vi "Main.vi"(11 "Module Admin":refnum<class "Delacor_lib_QMH_Module Admin.lvclass">) -> ()   [LabVIEW 2025, in "N4L_PSM3750_Interface.lvlib"]
doc: "This template is based from the Queued Message Handler design pattern and the Queued Message Handler Project Template that ships with LabVIEW 2014.\n\nThe main difference is that the Queue is private to this module and communication between modules is done via Broadcast and Request events.\n\nRequest events are wrapped via public API methods and are handled in the Event handler loop in this VI.\nAny module can register for Broadcast events sent by this module.\n\nThe Event Handling Loop generates messages based on user interface actions.\n\nThe Message Handling Loop processes messages generated by the Event Handling Loop, or by other messages. The messages are string values, so new messages can be added easily to the Message Cases case structure in the Message Handling Loop. Each message cluster can also provide an optional value for Message Data, which is a variant that can be converted to whatever message-specific data is required.\n_____\nBased on Delacor QMH Project Template 3.1.0.34.\n\n<b>Note:</b> This VI was modified by the <b>Validate DQMH Module</b> tool to wrap the FP.Open method in the module close code with a Conditional Disable Structure so it does not execute when the Main VI is running as a built EXE.\n\n<b>Note:</b> This VI was modified by the <b>Validate DQMH Module</b> tool to add a call to the Error Reported VI at the end of the 'Exit' MHL frame.\n\n<b>Note:</b> This VI was modified by the <b>Validate DQMH Module</b> tool to call the Release Message Queue VI in the top-level Error case."
uses:
  N4L_PSM3750_Interface.lvlib
  <vilib>/Delacor/Delacor QMH/Libraries/Module Admin_class/Delacor_lib_QMH_Module Admin.lvclass
  <vilib>/MGI/Panel Manager/Panel/Panel/Panel.lvclass
  <vilib>/Utility/miscctls.llb/LVPointTypeDef.ctl
  Module Data--cluster.ctl
  <vilib>/Delacor/Delacor QMH/Libraries/Message Queue_class/Delacor_lib_QMH_Message Queue.lvclass/Delacor_lib_QMH_Message Queue.ctl
  Stop Argument--cluster.ctl
  <vilib>/Delacor/Delacor QMH/Libraries/Module Admin_class/Delacor_lib_QMH_Module Admin.lvclass/Delacor_lib_QMH_Module Admin.ctl
  <vilib>/Delacor/Delacor QMH/Libraries/Message Queue_class/Delacor_lib_QMH_Enqueue Message (Single).vi
  <vilib>/Delacor/Delacor QMH/Libraries/Module Admin_class/Delacor_lib_QMH_Get External Launch.vi
  <vilib>/Utility/error.llb/Error Cluster From Error Code.vi
  <vilib>/ErrorRing/Error Ring.xnode
  <vilib>/Delacor/Delacor QMH/Libraries/Message Queue_class/Delacor_lib_QMH_Message Queue.lvclass
  <vilib>/MGI/Panel Manager/Panel/Panel Helper/Panel Helper.lvclass
  newtons4th-psm17xx-labview-files/NewtonsPSM1735.lvlib
panel:
  out "Connected?":bool
  in  "Panel":refnum<class "Panel.lvclass">
  in  "Simulate MHL Error":bool
  in  "Simulate EHL Error":bool
  out "error out":errorcluster
  out "Status":string
  # "This is a template that creates a DQMH Singleton using the MGI Panel Manager Framwork.\n\nImplement your user interface on this front panel. The Panel Manager Framework will manage showing and hiding the panel in the appropriate spot. \n\nSee the block diagram for more information on how to use this template."
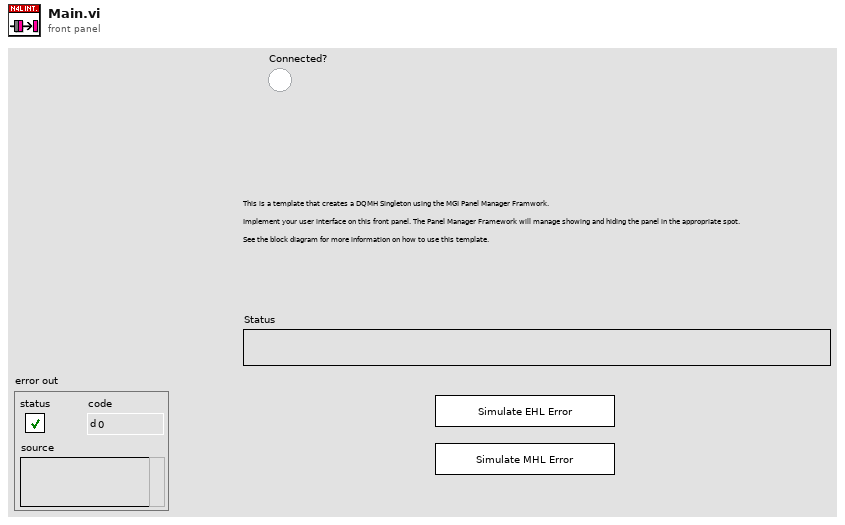
[diagram p1: front panel]
types:
  T1 = typedef "LVPointTypeDef.ctl" = cluster{"Horizontal":i16, "Vertical":i16}
  T2 = typedef "N4L_PSM3750_Interface.lvlib/Request Events--cluster.ctl" = cluster{"Stop Module":refnum<user-event>, "Show Panel":refnum<user-event>, "Hide Panel":refnum<user-event>, "Get Module Execution Status":refnum<user-event>, "Show Diagram":refnum<user-event>, "Change Panel":refnum<user-event>, "Initialise N4L Connection":refnum<user-event>, "Close N4L Connection":refnum<user-event>, "Reset N4L Instrument":refnum<user-event>, "Set Generator Configuration":refnum<user-event>, "Set Generator Output":refnum<user-event>, "Set Range":refnum<user-event>, "Set Trim Configuration":refnum<user-event>}
  T3 = typedef "Panel.lvlib/Panel Helper.lvclass/Panel Events.ctl" = cluster{"My Panel":refnum<user-event>, "Top Level Initialized":refnum<user-event>}
  T4 = typedef "N4L_PSM3750_Interface.lvlib/Module Data--cluster.ctl" = cluster{"Status":string, "State Map":map{string, dbl}}
  T5 = typedef "N4L_PSM3750_Interface.lvlib/Stop Argument--cluster.ctl" = cluster{"Origin":string, "Exit via Stop Module Req?":bool, "Wait for Module to stop?":bool}
  T6 = enum32{"invalid lock state", "Not Locked", "Locked (No Password)", "Password-protected"}
  T7 = typedef "N4L_PSM3750_Interface.lvlib/Initialise--cluster.ctl" = cluster{"VISA resource name":refnum<visa-resource-name>, "Baud Rate":u32, "ID Query":bool, "Reset":bool}
  T8 = typedef "N4L_PSM3750_Interface.lvlib/Generator Config--cluster.ctl" = cluster{"Waveform":enum16{"Sinewave", "Square"}, "Frequency (1000)":dbl, "Amplitude (2)":dbl, "Offset (0)":dbl}
  T9 = typedef "N4L_PSM3750_Interface.lvlib/Range Config--cluster.ctl" = cluster{"Input Ranging Mode (Auto)":enum16{"AUTO", "UPAUTO", "1mV", "3mV", "10mV", "30mV", "100mV", "300mV", "1V", "3V", "10V"}, "Input Input Type (Internal)":u16, "Input Selection (CH1)":enum16{"CH1", "CH2"}, "Input Connection (Main) ":u16, "Input Coupling (Internal)":enum16{"AC+DC", "AC"}, "Input Shunt Value (0,02)":dbl, "Input Voltage Scale factor (1)":dbl}
  T10 = enum16{"AUTO", "UPAUTO", "1mV", "3mV", "10mV", "30mV", "100mV", "300mV", "1V", "3V", "10V"}
  T11 = cluster{"AC Trim Data (Disabled)":u16, "AC Level (1)":dbl, "Tolerance (10)":dbl}
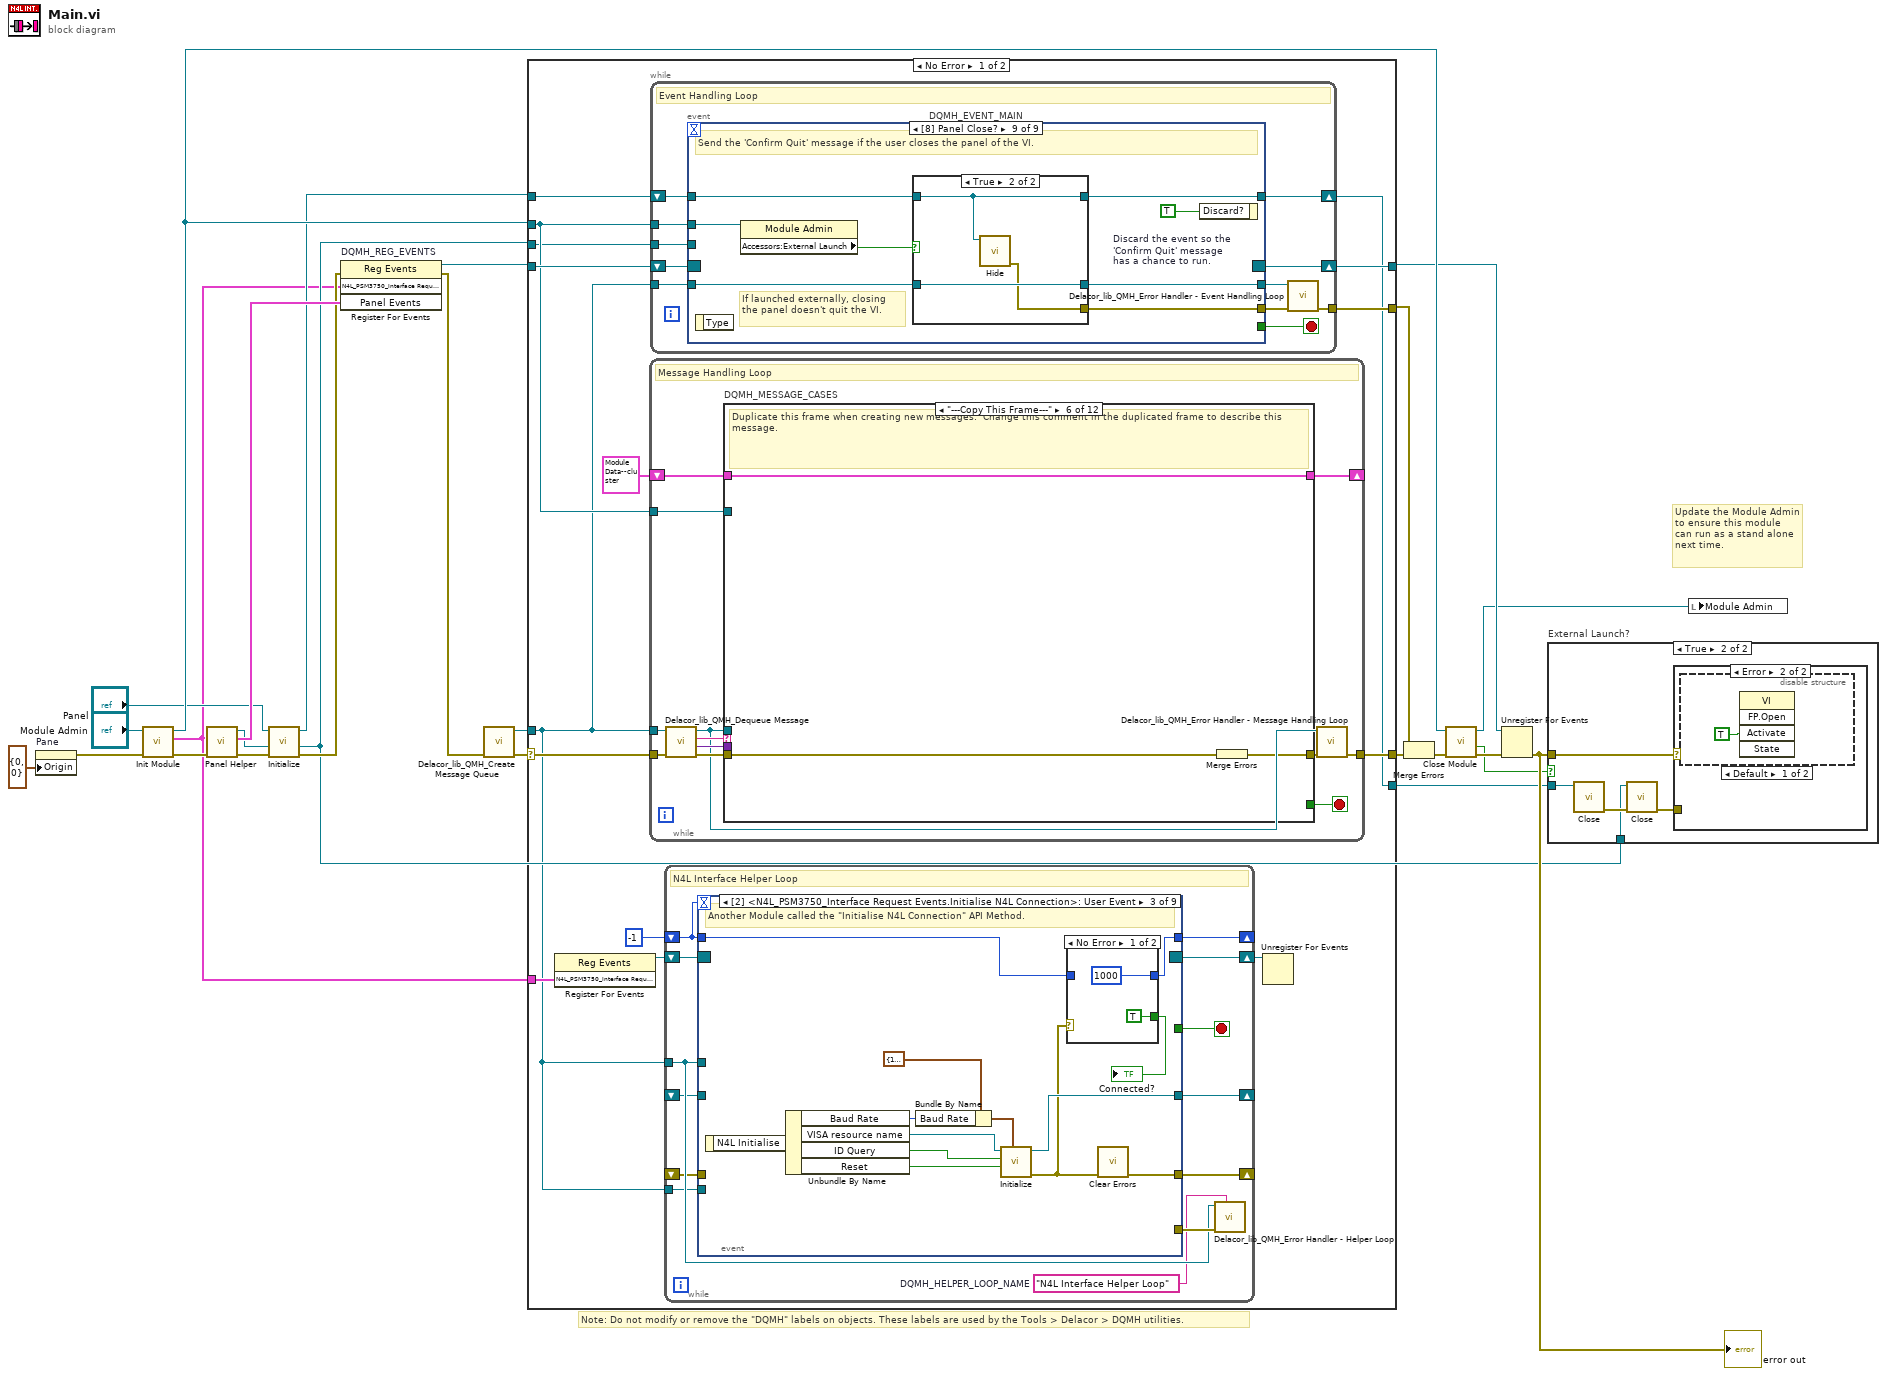
[diagram p0: block diagram]
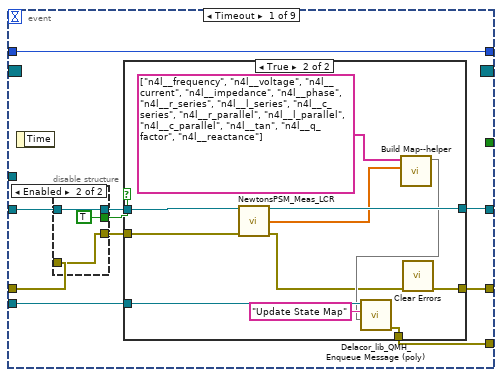
[diagram p5: hidden frame]
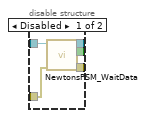
[diagram p6: hidden frame]
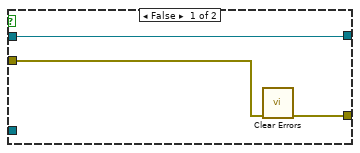
[diagram p7: hidden frame]
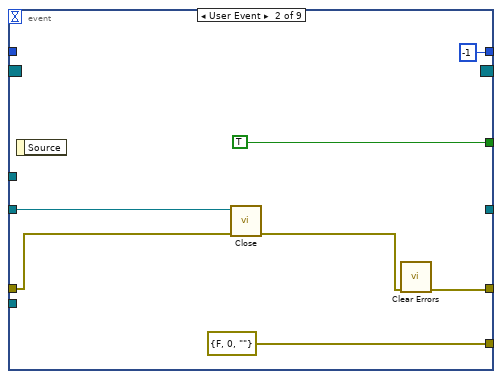
[diagram p8: hidden frame]
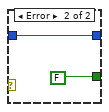
[diagram p9: hidden frame]
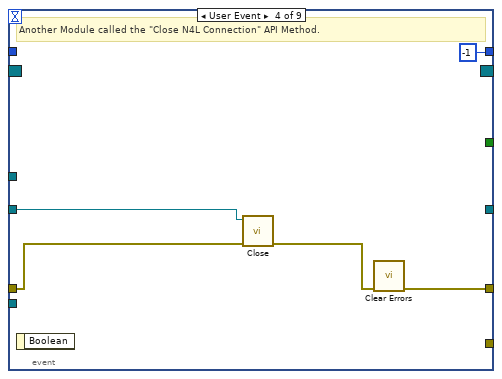
[diagram p10: hidden frame]
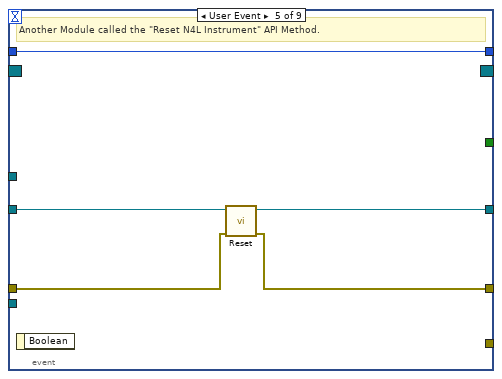
[diagram p11: hidden frame]
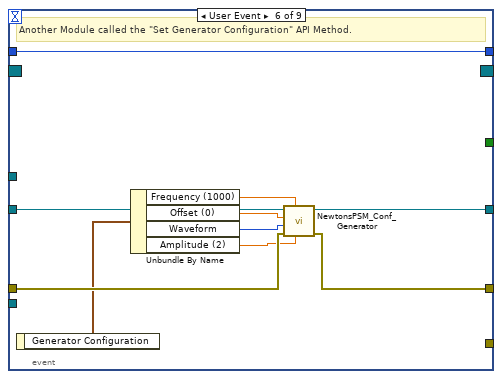
[diagram p12: hidden frame]
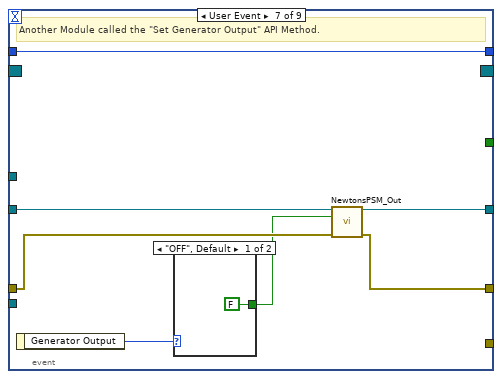
[diagram p13: hidden frame]
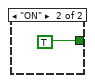
[diagram p14: hidden frame]
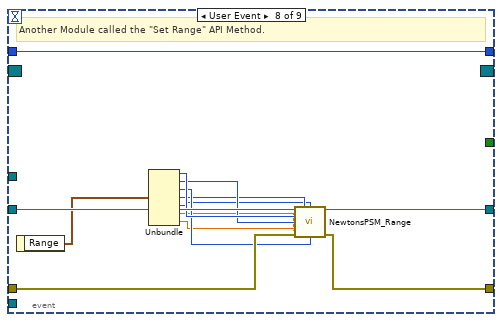
[diagram p15: hidden frame]
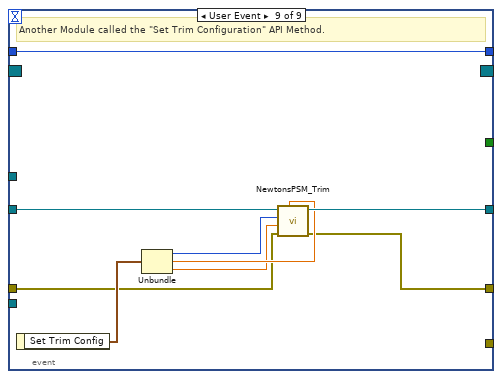
[diagram p16: hidden frame]
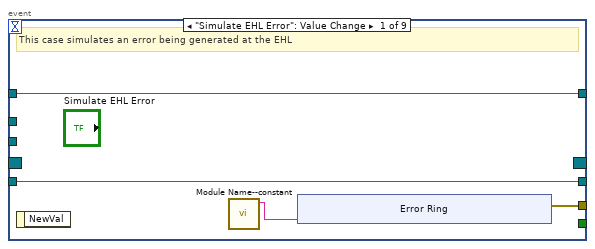
[diagram p17: hidden frame]
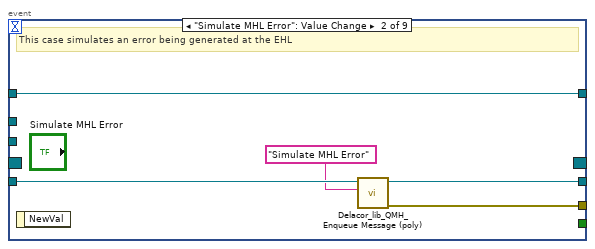
[diagram p18: hidden frame]
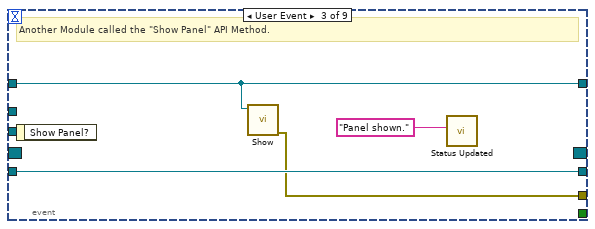
[diagram p19: hidden frame]
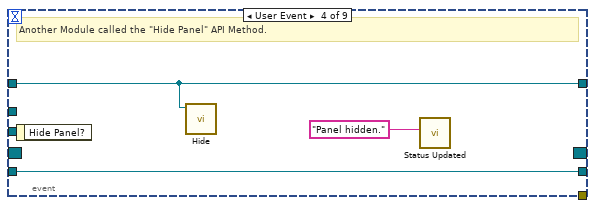
[diagram p20: hidden frame]
diagram:
  # "Note: Do not modify or remove the \"DQMH\" labels on objects. These labels are used by the Tools > Delacor > DQMH utilities."
  # "Update the Module Admin to ensure this module can run as a stand alone next time."
  n1 = property on="Pane" class="Pane"("Origin"=T1 {"Horizontal"=0, "Vertical"=0}) -> (error out=w2:errorcluster)  [unwired: 2 in, 1 out]
  n2 = call "Init Module.vi"("error in (no error)"=w2, "Singleton Module Admin in"="Module Admin") -> ("error out"=w12:errorcluster, "N4L_PSM3750_Interface Request Events"=w1:T2, "Singleton Module Admin out"=w26:refnum<class "Delacor_lib_QMH_Module Admin.lvclass">)  [unwired: 7 in]
  n3 = call <vilib>:"Panel Helper.vi"("Error In"=w12) -> ("Error Out"=w9:errorcluster, "Panel Events"=w11:T3, "Panel Helper out"=w8:refnum<class "Panel Helper.lvclass">)  [unwired: 8 in]
  n4 = call <vilib>:"Initialize.vi"("error in (no error)"=w9, "My Helper in"=w8, "Panel In"="Panel") -> ("error out"=w6:errorcluster, "My Helper out"=w5:refnum<class "Panel Helper.lvclass">, "Panel Out"=w4:refnum<class "Panel.lvclass">)  [unwired: 6 in]
  n5 = register-events "DQMH_REG_EVENTS"(error in=w6, w1, w11) -> (reference out=w23:refnum<event-registration>, error out=w10:errorcluster)  [unwired: 1 in]
  n6 = call <vilib>:"Delacor_lib_QMH_Create Message Queue.vi"("error in"=w10) -> ("error out"=w14:errorcluster, "Message Queue"=w22:refnum<class "Delacor_lib_QMH_Message Queue.lvclass">)  [unwired: 9 in]
  n7 = case shown="No Error" w14 {
    selector: w14 -> [w36 w378]
    tunnel: [w41 w378] -> w25
    tunnel: [w40 w383] -> w24
    tunnel: w23 -> [w38 w383]
    tunnel: w22 -> [w27 w374]
    tunnel: [w37 _] -> w18
    tunnel: w26 -> [w35 w379]
    tunnel: w4 -> [w33 w375]
    tunnel: w5 -> [w34 _]
    tunnel: [w32 w375] -> w13
    tunnel: w1 -> [w31 _]
    frame No Error {
      n8 = register-events ("DQMH_HELPER_REGFOREVENTS")(w31) -> (reference out=w29:refnum<event-registration>)  [unwired: 2 in, 1 out]
      n9 = while {
        tunnel: w27 -> [w246]
        shift-right: [w252] -> _
        shift-left: T4 {"Status"="", "State Map"={}} ("Data Cluster") -> [w253]
        tunnel: w36 -> [w250]
        tunnel: [w244] -> w41
        tunnel: w35 -> [w243]
        stop <- w251 stop-if-true
        # "Message Handling Loop"
        n10 = call-dynamic "Delacor_lib_QMH_Dequeue Message.vi"("error in"=w250, "Message Queue in"=w246) -> ("error out"=w249:errorcluster, "Message Data"=w247:variant, "Message"=w248:string, "Message Queue out"=w245:refnum<class "Delacor_lib_QMH_Message Queue.lvclass">)  [unwired: 6 in]
        n11 = case "DQMH_MESSAGE_CASES" shown="\"---Copy This Frame---\"" w248 {
          selector: w248 -> [_ _ _ _ _ _ _ _ _ _ _ w363]
          tunnel: w245 -> [_ _ _ _ _ _ _ _ w328 w343 w359 _]
          tunnel: w249 -> [w257 w269 w273 w291 w301 w309 w312 w317 w334 w347 w361 _]
          tunnel: [w258 w270 w272 w289 w297 w307 w310 w315 w325 w345 w355 w364] -> w254
          tunnel: w253 -> [w263 w271 w274 w290 w296 w308 w311 w316 w333 w346 w358 w365]
          tunnel: [w262 w271 w274 w290 w295 w308 w311 w316 w333 w346 w358 w365] -> w252
          tunnel: [_ _ _ _ _ _ _ _ _ _ w357 _] -> w251
          tunnel: w247 -> [_ w268 _ _ w300 _ _ _ w332 _ w354 _]
          tunnel: w243 -> [w255 _ _ _ _ _ _ _ w327 _ w348 _]
          frame "Initialize" {
            w261 = "Initial Message" ("Initial Message")
            # "#CodeNeeded - Initialize the appearance of the front panel."
            # "#CodeNeeded - Initialize your state data here."
            # "Initialize - Any operation that needs to be done before the module can receive messages. Synchronize Caller Events.vi will inform Start Module.vi that the module has launched and is ready to receive messages. Module Did Init.vi will broadcast that the module initialized."
            n12 = call "Synchronize Caller Events.vi"("error in (no error)"=w257, "Singleton Module Admin in"=w255) -> ("error out"=w256:errorcluster)  [unwired: 8 in, 1 out]
            n13 = Bundle By Name(cluster=w263, "Status"=w261) -> (w262:T4)
            n14 = local write "Status"(w261) -> ()
            n15 = call "Module Name--constant.vi"() -> ("Module Name"=w259:string)  [unwired: 11 in]
            n16 = call "Module Did Init.vi"("error in (no error)"=w256, "Initialized?"=TRUE, "Origin"=w259) -> ("error out"=w258:errorcluster)  [unwired: 8 in]
          }
          frame "Update Display" {
            # "Broadcast updated status to any VI registered to listen to this module's broadcast events."
            # "Convert the message data to a string to display in the Status indicator."
            # "#CodeRecommended - If you wish to decouple the Message Handling Loop from your user interface, consider creating User Events (like the \"Stop\" event in this VI) to message the Event Handling Loop whenever the user interface needs updating."
            # "Update Display - Update user interface here."
            n17 = Variant To Data(error in=w269, type="" ("Empty String Constant"), Variant=w268) -> (data=w266:string, error out=w265:errorcluster)
            "Status" <- w266
            n18 = call "Status Updated.vi"("error in (no error)"=w265, "Status"=w266) -> ("error out"=w264:errorcluster)  [unwired: 9 in]
            n19 = Merge Errors(w264) -> (w270:errorcluster)
          }
          frame "Show Diagram" {
            # "Show Diagram - Show the block diagram of this VI. Used as a debugging tool. There is a button in the module tester that fires the Show Diagram request, which runs this message. Note that the diagram will not be displayed if it is password-protected and the password is not in the cache."
            n20 = disable-structure shown="RUN_TIME_ENGINE==False" {
              disable-tunnel: [w282 w288] -> w272
              disable-tunnel: w273 -> [w281 w288]
              frame condition #0 (active) {
                # "functionality not available in exe"
                n21 = invoke class="VI" method="Lock State.Get"(error in=w281) -> (error out=w280:errorcluster, "Get Lock State"=w279:T6, "pwd in cache"=w276:bool)  [unwired: 3 in, 1 out]
                n22 = Equal?(x=T6."Password-protected", y=w279) -> (x = y?=w277:bool)
                n23 = Compound Arithmetic op=AND(w277, invert w276) -> (w275:bool)
                n24 = case shown="False" w275 {
                  tunnel: [w285 w287] -> w282
                  tunnel: w280 -> [w283 w287]
                  frame False {
                    n25 = property class="VI"(error in=w283, "BDWin.Open"=TRUE ("Block Diagram Window:Open")) -> (error out=w285:errorcluster)  [unwired: 1 in, 1 out]
                    n26 = call "Status Updated.vi"("Status"="Block Diagram shown." ("format string")) -> ()  [unwired: 10 in, 1 out]
                  }
                  frame True {
                    # "Password-protected VI, and the password is not in the cache. Do not show the diagram."
                  }
                }
              }
              frame condition #1 {
              }
            }
          }
          frame "--- Module Specific ---" {
            # "Separator -- The following cases handle messages specific to this Module."
            n27 = Merge Errors(w291) -> (w289:errorcluster)
          }
          frame "Update State Map" {
            w299 = map{string, dbl} {}  # Size: 0
            n28 = Variant To Data(error in=w301, type=w299, Variant=w300) -> (data=w294:map{string, dbl}, error out=w298:errorcluster)
            n29 = Unbundle By Name(w296) -> ("State Map"=w293:map{string, dbl})
            n30 = for {
              tunnel: w294 -> [w304] mode=indexing
              shift-right: [w305] -> w292
              shift-left: w293 -> [w306]
              n31 = Unbundle(w304) -> (w303:string, w302:dbl)
              n32 = Insert Into Map(map in=w306, key=w303, value=w302) -> (map out=w305:map{string, dbl})  [unwired: 2 out]
            }
            n33 = Bundle By Name(cluster=w296, "State Map"=w292) -> (w295:T4)
            n34 = call "Broadcast State.vi"("error in"=w298, "State Map"=w292) -> ("error out"=w297:errorcluster)  [unwired: 9 in]
          }
          frame "---Copy This Frame---" {
            # "Duplicate this frame when creating new messages.  Change this comment in the duplicated frame to describe this message."
            n35 = Merge Errors(w309) -> (w307:errorcluster)
          }
          frame "--- Exit and Error Handling---" {
            # "Separator - The following cases handle errors and exit messages."
            n36 = Merge Errors(w312) -> (w310:errorcluster)
          }
          frame "Simulate MHL Error" {
            # "Simulate an error occurring at the MHL"
            n37 = call "Module Name--constant.vi"() -> ("Module Name"=w314:string)  [unwired: 11 in]
            n38 = xnode "Error Ring"("parameter 0"=w314) -> ("error out"=w313:errorcluster)
            n39 = Merge Errors(w317, w313) -> (w315:errorcluster)
          }
          frame "Error" {
            # "#CodeRecommended - If you ever change the name of this \"Error\" message, you'll need to update the name in the Check Loop Error.vi as well."
            # "#CodeRecommended - If the module is running in standalone mode (External Launch = FALSE), this code will pop up an error dialog and call the 'Exit' message if an error occurs. Add more fine-grained error handling here."
            # "Error - Check the error message data and respond accordingly. This message is sent by the \"Error Handler\" VIs at the end of each loop in this application."
            n40 = property class="Module Admin"(reference=w327) -> ("Accessors:External Launch"=w326:bool)  [unwired: 1 in, 2 out]
            n41 = Variant To Data(error in=w334, type=errorcluster {"status"=FALSE, "code"=0, "source"=""} ("error constant"), Variant=w332) -> (data=w335:errorcluster, error out=w330:errorcluster)
            n42 = call "Error Reported.vi"("Error"=w335) -> ()  [unwired: 10 in, 1 out]
            n43 = case shown="False" w326 {
              tunnel: [w340 _] -> w329
              tunnel: w328 -> [w339 _]
              tunnel: w335 -> [w336 _]
              frame False {
                # "If the module is running standalone, then pop up an error dialog and call the \"Exit\" message."
                n44 = call <vilib>:"Simple Error Handler.vi"("error in (no error)"=w336) -> ()  [unwired: 4 in, 5 out]
                n45 = call-poly <vilib>:"Delacor_lib_QMH_Enqueue Message (poly).vi"("Priority Message? (F)"=TRUE, "Message"="Exit", "Message Queue in"=w339) -> ("error out"=w340:errorcluster)  [unwired: 7 in, 1 out]
              }
              frame True {
                # "If the module was launched externally, calling the Error Reported broadcast VI is the only action performed by the \"Error\" message. The module's caller can then process the error appropriately."
              }
            }
            n46 = Merge Errors(w330, w329) -> (w325:errorcluster)
            n47 = local write "error out"(w325) -> ()
          }
          frame "Confirm Quit" {
            # "#CodeNeeded - If you want to provide an \"Are you sure\" dialog (or some other notification) before the application exits, place that code here. This message is typically sent from a Panel Close? event."
            # "Confirm Quit - Message that can confirm whether or not the user wants to exit the application."
            n48 = call-poly <vilib>:"Delacor_lib_QMH_Enqueue Message (poly).vi"("Priority Message? (F)"=TRUE, "error in"=w347, "Message"="Exit", "Message Queue in"=w343) -> ("error out"=w344:errorcluster)  [unwired: 6 in, 1 out]
            n49 = Merge Errors(w344) -> (w345:errorcluster)
          }
          frame "Exit" {
            w352 = 91  # 91: not all Exit messages will have an argument
            w357 = TRUE  # Stop the VI
            # "Release the message queue reference"
            # "#CodeNeeded - Add any required cleanup code here"
            # "Exit - Exit the application."
            n50 = Variant To Data(error in=w361, type=T5 {"Origin"="", "Exit via Stop Module Req?"=FALSE, "Wait for Module to stop?"=FALSE} ("Stop Argument"), Variant=w354) -> (data=w350:T5, error out=w353:errorcluster)
            n51 = call <vilib>:"Clear Errors.vi"("error in (no error)"=w353, "specific error code to clear (0: all)"=w352) -> ("error out"=w360:errorcluster)  [unwired: 4 in, 1 out]
            n52 = call-dynamic "Delacor_lib_QMH_Release Message Queue.vi"("error in"=w360, "Message Queue"=w359) -> ("error out"=w356:errorcluster)  [unwired: 9 in]
            n53 = call "Handle Exit.vi"("Stop Argument"=w350, "Admin in"=w348) -> ("error out"=w349:errorcluster)  [unwired: 8 in, 1 out]
            n54 = Merge Errors(w349, w356) -> (w355:errorcluster)
            n55 = call "Error Reported.vi"("Error"=w355) -> ()  [unwired: 10 in, 1 out]
          }
          frame Default {
            # "'Default' case only runs if there is a message that isn't defined in any of the other cases.  Output a programming error."
            n56 = call "Module Name--constant.vi"() -> ("Module Name"=w362:string)  [unwired: 11 in]
            n57 = xnode "Error Ring"("parameter 0"=w363, "parameter 1"=w362) -> ("error out"=w364:errorcluster)
          }
        }
        n58 = call-dynamic "Delacor_lib_QMH_Error Handler - Message Handling Loop.vi"("error in"=w254, "Message Queue in"=w245) -> ("dup error in"=w244:errorcluster)  [unwired: 8 in, 1 out]
      }
      n59 = while {
        tunnel: w27 -> [w172]
        shift-right: [w170] -> w40
        shift-left: w38 -> [w171]
        tunnel: [w166] -> w37
        tunnel: w35 -> [w165]
        tunnel: w34 -> [w164]
        shift-right: [w162] -> w32
        shift-left: w33 -> [w163]
        stop <- w168 stop-if-true
        # "Event Handling Loop"
        n60 = event "DQMH_EVENT_MAIN" shown="[8] Panel Close?" {
          selector: w171 -> [_ _ _ _ _ _ _ _ _]
          dyn-events: [_ _ _ _ _ _ _ _ _] -> w170
          timeout: _ -> [_ _ _ _ _ _ _ _ _]
          tunnel: [_ _ _ _ _ _ TRUE ("Discard?") _ _] -> w168
          tunnel: w172 -> [w176 w188 w192 w195 w199 w204 w216 w226 w233]
          tunnel: [w175 w185 w190 _ w198 w201 w210 w222 w232] -> w169
          tunnel: [w176 w187 w192 w195 w199 w203 w215 w226 w231] -> w167
          tunnel: w165 -> [_ _ _ _ _ _ _ _ w230]
          tunnel: w164 -> [_ _ _ _ _ _ _ w221 _]
          tunnel: w163 -> [w173 w184 w191 w194 w196 w200 w205 w225 w228]
          tunnel: [w173 w184 w191 w194 w196 w200 w205 w220 w227] -> w162
          event "Simulate EHL Error": Value Change {
            # "This case simulates an error being generated at the EHL"
            n61 = event-data() -> ()  [unwired: 1 in, 1 out]
            n62 = call "Module Name--constant.vi"() -> ("Module Name"=w174:string)  [unwired: 11 in]
            n63 = xnode "Error Ring"("parameter 0"=w174) -> ("error out"=w175:errorcluster)
          }
          event "Simulate MHL Error": Value Change {
            # "This case simulates an error being generated at the EHL"
            n64 = event-data() -> ()  [unwired: 1 in, 1 out]
            n65 = call-poly <vilib>:"Delacor_lib_QMH_Enqueue Message (poly).vi"("Message"="Simulate MHL Error", "Message Queue in"=w188) -> ("error out"=w185:errorcluster, "Message Queue out"=w187:refnum<class "Delacor_lib_QMH_Message Queue.lvclass">)  [unwired: 8 in]
          }
          event User Event {
            # "Another Module called the \"Show Panel\" API Method."
            n66 = event-data() -> ()  [unwired: 1 in, 1 out]
            n67 = call <vilib>:"Show.vi"("Panel in"=w191) -> ("Error Out"=w190:errorcluster)  [unwired: 10 in]
            n68 = call "Status Updated.vi"("Status"="Panel shown." ("format string")) -> ()  [unwired: 10 in, 1 out]
          }
          event User Event {
            # "Another Module called the \"Hide Panel\" API Method."
            n69 = event-data() -> ()  [unwired: 1 in, 1 out]
            n70 = call <vilib>:"Hide.vi"("Panel In"=w194) -> ()  [unwired: 10 in, 1 out]
            n71 = call "Status Updated.vi"("Status"="Panel hidden." ("format string")) -> ()  [unwired: 10 in, 1 out]
          }
          event User Event {
            # "Another Module called the \"Get Module Execution Status\" API Method."
            n72 = event-data() -> ()  [unwired: 1 in, 1 out]
            n73 = call "Update Module Execution Status.vi"("Running?"=TRUE) -> ("error out"=w198:errorcluster)  [unwired: 10 in]
          }
          event User Event {
            # "Another Module called the \"Show Diagram\" API Method."
            n74 = event-data() -> ()  [unwired: 1 in, 1 out]
            n75 = call-poly <vilib>:"Delacor_lib_QMH_Enqueue Message (poly).vi"("Message"="Show Diagram", "Message Queue in"=w204) -> ("error out"=w201:errorcluster, "Message Queue out"=w203:refnum<class "Delacor_lib_QMH_Message Queue.lvclass">)  [unwired: 8 in]
          }
          event User Event {
            # "The Stop Module Event can get fired from the Exit message in the MHL. The queue gets destroyed in that case. If the queue no longer exists, the Enqueue Exit as a priority message will return error 1. It is safe to ignore, because the module is already exiting."
            # "Another Module called the \"Stop Module\" API Method  or the Message Handling Loop below."
            n76 = event-data() -> ("Origin"=w214:string, "Exit via Stop Module Req?"=w208:bool, "Wait for Module to stop?"=w207:bool)  [unwired: 1 in]
            n77 = call <vilib>:"Hide.vi"("Panel In"=w205) -> ()  [unwired: 10 in, 1 out]
            n78 = local write "Status"(w214) -> ()
            n79 = Bundle By Name(cluster=T5 {"Origin"="", "Exit via Stop Module Req?"=FALSE, "Wait for Module to stop?"=FALSE} ("Stop Argument"), "Exit via Stop Module Req?"=w208, "Wait for Module to stop?"=w207) -> (w206:T5)
            n80 = call-poly <vilib>:"Delacor_lib_QMH_Enqueue Message (poly).vi"("Priority Message? (F)"=TRUE, "Message Data"=w206, "Message"="Exit", "Message Queue in"=w216) -> ("error out"=w211:errorcluster, "Message Queue out"=w215:refnum<class "Delacor_lib_QMH_Message Queue.lvclass">)  [unwired: 6 in]
            n81 = call <vilib>:"Clear Errors.vi"("error in (no error)"=w211, "specific error code to clear (0: all)"=1) -> ("error out"=w210:errorcluster)  [unwired: 4 in, 1 out]
          }
          event User Event {
            # "Another Module called the \"Change Panel\" API Method."
            n82 = event-data() -> ("New Panel"=w224:refnum<class "Panel.lvclass">)  [unwired: 1 in]
            n83 = call-dynamic <vilib>:"Close.vi"("Panel In"=w225) -> ("Error Out"=w223:errorcluster)  [unwired: 10 in]
            n84 = call <vilib>:"Initialize.vi"("error in (no error)"=w223, "My Helper in"=w221, "Panel In"=w224) -> ("error out"=w222:errorcluster, "Panel Out"=w220:refnum<class "Panel.lvclass">)  [unwired: 6 in, 1 out]
            n85 = call "Status Updated.vi"("Status"="Panel changed.") -> ()  [unwired: 10 in, 1 out]
          }
          event Panel Close? {
            w234 = TRUE  # Discard the event so the 'Confirm Quit' message has a chance to run.
            # "If launched externally, closing the panel doesn't quit the VI."
            # "Send the 'Confirm Quit' message if the user closes the panel of the VI."
            n86 = event-data() -> ()  [unwired: 1 in, 1 out]
            n87 = property class="Module Admin"(reference=w230) -> ("Accessors:External Launch"=w229:bool)  [unwired: 1 in, 2 out]
            n88 = case shown="True" w229 {
              tunnel: w233 -> [w239 w242]
              tunnel: [w238 w240] -> w232
              tunnel: [w237 w242] -> w231
              tunnel: w228 -> [w235 w241]
              tunnel: [w235 w241] -> w227
              frame False {
                n89 = call-poly <vilib>:"Delacor_lib_QMH_Enqueue Message (poly).vi"("Message"="Confirm Quit", "Message Queue in"=w239) -> ("error out"=w238:errorcluster, "Message Queue out"=w237:refnum<class "Delacor_lib_QMH_Message Queue.lvclass">)  [unwired: 8 in]
              }
              frame True {
                n90 = call <vilib>:"Hide.vi"("Panel In"=w241) -> ("Error Out"=w240:errorcluster)  [unwired: 10 in]
              }
            }
            n91 = event-data("Discard?"=w234) -> ()  [unwired: 1 in, 1 out]
          }
        }
        n92 = call-dynamic "Delacor_lib_QMH_Error Handler - Event Handling Loop.vi"("error in"=w169, "Message Queue in"=w167) -> ("dup error in"=w166:errorcluster)  [unwired: 8 in, 1 out]
      }
      n93 = while "DQMH_HELPER_LOOP" {
        shift-right: [w54] -> _
        shift-left: -1 -> [w53]
        shift-right: [w51] -> w30
        shift-left: w29 -> [w52]
        tunnel: w27 -> [w48]
        shift-right: [w46] -> _
        shift-left: _ -> [w45]
        shift-right: [w44] -> _
        shift-left: _ -> [w43]
        tunnel: w27 -> [w42]
        stop <- w50 stop-if-true
        w47 = "N4L Interface Helper Loop"  # DQMH_HELPER_LOOP_NAME
        # "N4L Interface Helper Loop"
        n94 = event "DQMH_HELPER_EVENT_STRUCTURE" shown="[2] <N4L_PSM3750_Interface Request Events.Initialise N4L Connection>: User Event" {
          selector: w52 -> [_ _ _ _ _ _ _ _ _]
          dyn-events: [_ _ _ _ _ _ _ _ _] -> w51
          timeout: w53 -> [_ _ _ _ _ _ _ _ _]
          tunnel: w53 -> [w64 _ w98 _ w120 w130 w137 w152 w161]
          tunnel: [w64 -1 w97 -1 w120 w130 w137 w152 w161] -> w54
          tunnel: [_ TRUE _ _ _ _ _ _ _] -> w50
          tunnel: [w57 errorcluster {"status"=FALSE, "code"=0, "source"=""} ("error constant") _ _ _ _ _ _ _] -> w49
          tunnel: w48 -> [_ _ _ _ _ _ _ _ _]
          tunnel: [w56 w88 w95 w111 w117 w127 w134 w148 w153] -> w46
          tunnel: w45 -> [w62 w90 _ w114 w116 w126 w133 w149 w154]
          tunnel: [w59 _ w99 _ w118 w128 w135 w150 w159] -> w44
          tunnel: w43 -> [w63 w91 _ w115 w119 w129 w136 w151 w160]
          tunnel: w42 -> [w58 _ _ _ _ _ _ _ _]
          event Timeout {
            n95 = event-data() -> ()  [unwired: 1 in, 1 out]
            n96 = disable-structure shown="Enabled" {
              disable-tunnel: w63 -> [w69 w72]
              disable-tunnel: w62 -> [w68 w70]
              disable-tunnel: [w67 w72] -> w61
              disable-tunnel: [w66 w70] -> w60
              disable-tunnel: [w65 TRUE ("Data Available")] -> w55
              frame Disabled {
                n97 = call "NewtonsPSM_WaitData.vi"("error in (no error)"=w68, "VISA session"=w69) -> ("error out"=w66:errorcluster, "Data Available"=w65:bool, "dup VISA session"=w67:refnum<visa-resource-name>)  [unwired: 5 out]
              }
              frame Enabled {
              }
            }
            n98 = case shown="True" w55 {
              tunnel: w61 -> [w75 w86]
              tunnel: w60 -> [w73 w85]
              tunnel: [w75 w84] -> w59
              tunnel: w58 -> [_ w81]
              tunnel: [_ w80] -> w57
              tunnel: [w74 w76] -> w56
              frame False {
                n99 = call <vilib>:"Clear Errors.vi"("error in (no error)"=w73) -> ("error out"=w74:errorcluster)  [unwired: 5 in, 1 out]
              }
              frame True {
                n100 = call "NewtonsPSM_Meas_LCR.vi"("VISA session"=w86, "error in (no error)"=w85) -> ("dup VISA session"=w84:refnum<visa-resource-name>, "Measure"=w83:dbl[], "error out"=w77:errorcluster)  [unwired: 10 in, 1 out]
                n101 = call "Build Map--helper.vi"("Measure"=w83, "Array"=string[] ["n4l__frequency", "n4l__voltage", "n4l__current", "n4l__impedance", "n4l__phase", "n4l__r_series", "n4l__l_series", "n4l__c_series", "n4l__r_parallel", "n4l__l_parallel", "n4l__c_parallel", "n4l__tan", "n4l__q_factor", "n4l__reactance"]) -> ("Map"=w78:map{string, dbl})  [unwired: 9 in]
                n102 = call-poly <vilib>:"Delacor_lib_QMH_Enqueue Message (poly).vi"("Message Data"=w78, "Message"="Update State Map", "Message Queue in"=w81) -> ("error out"=w80:errorcluster)  [unwired: 7 in, 1 out]
                n103 = call <vilib>:"Clear Errors.vi"("error in (no error)"=w77) -> ("error out"=w76:errorcluster)  [unwired: 5 in, 1 out]
              }
            }
          }
          event User Event {
            n104 = event-data() -> ()  [unwired: 1 in, 1 out]
            n105 = call <vilib>:"Close.vi"("error in (no error)"=w90, "VISA resource name"=w91) -> ("error out"=w87:errorcluster)  [unwired: 9 out]
            n106 = call <vilib>:"Clear Errors.vi"("error in (no error)"=w87) -> ("error out"=w88:errorcluster)  [unwired: 5 in, 1 out]
          }
          event User Event {
            # "Another Module called the \"Initialise N4L Connection\" API Method."
            n107 = event-data() -> ("N4L Initialise"=w106:T7)  [unwired: 1 in]
            n108 = Unbundle By Name(w106) -> ("Baud Rate"=w103:u32, "VISA resource name"=w105:refnum<visa-resource-name>, "ID Query"=w101:bool, "Reset"=w100:bool)
            n109 = Bundle By Name(cluster=cluster{"Baud Rate":u32} {"Baud Rate"=19200} ("Serial Configuration"), "Baud Rate"=w103) -> (w102:cluster{"Baud Rate":u32})
            n110 = call <vilib>:"Initialize.vi"("Serial Configuration"=w102, "Reset (True)"=w100, "ID Query (True)"=w101, "VISA resource name"=w105) -> ("error out"=w96:errorcluster, "VISA resource name out"=w99:refnum<visa-resource-name>)  [unwired: 6 in]
            n111 = case shown="No Error" w96 {
              tunnel: w98 -> [_ w110]
              tunnel: [1000 w110] -> w97
              tunnel: [TRUE FALSE] -> w94
              frame No Error {
              }
              frame Error {
              }
            }
            "Connected?" <- w94
            n112 = call <vilib>:"Clear Errors.vi"("error in (no error)"=w96) -> ("error out"=w95:errorcluster)  [unwired: 5 in, 1 out]
          }
          event User Event {
            # "Another Module called the \"Close N4L Connection\" API Method."
            n113 = event-data() -> ()  [unwired: 1 in, 1 out]
            n114 = call <vilib>:"Close.vi"("error in (no error)"=w114, "VISA resource name"=w115) -> ("error out"=w112:errorcluster)  [unwired: 9 in]
            n115 = call <vilib>:"Clear Errors.vi"("error in (no error)"=w112) -> ("error out"=w111:errorcluster)  [unwired: 5 in, 1 out]
          }
          event User Event {
            # "Another Module called the \"Reset N4L Instrument\" API Method."
            n116 = event-data() -> ()  [unwired: 1 in, 1 out]
            n117 = call "Reset.vi"("error in (no error)"=w116, "VISA resource name"=w119) -> ("error out"=w117:errorcluster, "VISA resource name out"=w118:refnum<visa-resource-name>)  [unwired: 8 in]
          }
          event User Event {
            # "Another Module called the \"Set Generator Configuration\" API Method."
            n118 = event-data() -> ("Generator Configuration"=w125:T8)  [unwired: 1 in]
            n119 = Unbundle By Name(w125) -> ("Frequency (1000)"=w121:dbl, "Offset (0)"=w122:dbl, "Waveform"=w124:enum16{"Sinewave", "Square"}, "Amplitude (2)"=w123:dbl)
            n120 = call "NewtonsPSM_Conf_Generator.vi"("Amplitude (2)"=w123, "Frequency (1000)"=w121, "error in"=w126, "Waveform (Sinewave)"=w124, "Offset (0)"=w122, "VISA.name"=w129) -> ("error out"=w127:errorcluster, "VISA.name out"=w128:refnum<visa-resource-name>)  [unwired: 4 in]
          }
          event User Event {
            # "Another Module called the \"Set Generator Output\" API Method."
            n121 = event-data() -> ("Generator Output"=w132:enum16{"OFF", "ON"})  [unwired: 1 in]
            n122 = case shown="\"OFF\", Default" w132 {
              tunnel: [FALSE TRUE] -> w131
              frame "OFF", Default {
              }
              frame "ON" {
              }
            }
            n123 = call "NewtonsPSM_Out.vi"("VISA session"=w136, "Output (F: OFF)"=w131, "error in (no error)"=w133) -> ("dup VISA session"=w135:refnum<visa-resource-name>, "error out"=w134:errorcluster)  [unwired: 11 in]
          }
          event User Event {
            # "Another Module called the \"Set Range\" API Method."
            n124 = event-data() -> ("Range"=w147:T9)  [unwired: 1 in]
            n125 = Unbundle(w147) -> ("Input Ranging Mode (Auto)"=w146:T10, "Input Input Type (Internal)"=w145:u16, "Input Selection (CH1)"=w144:enum16{"CH1", "CH2"}, "Input Connection (Main)"=w143:u16, "Input Coupling (Internal)"=w142:enum16{"AC+DC", "AC"}, "Input Shunt Value (0,02)"=w140:dbl, "Input Voltage Scale factor (1)"=w141:dbl)
            n126 = call "NewtonsPSM_Range.vi"("VISA session"=w151, "Input Connection (Main)"=w143, "Input Coupling (Internal)"=w142, "Input Ranging Mode (Auto)"=w146, "Input Input Type (Internal)"=w145, "Input Voltage Scale factor (1)"=w141, "error in (no error)"=w149, "Input Shunt Value (0,02)"=w140, "Input Selection (CH1)"=w144) -> ("dup VISA session"=w150:refnum<visa-resource-name>, "error out"=w148:errorcluster)  [unwired: 5 in]
          }
          event User Event {
            # "Another Module called the \"Set Trim Configuration\" API Method."
            n127 = event-data() -> ("Set Trim Config"=w158:T11)  [unwired: 1 in]
            n128 = Unbundle(w158) -> ("AC Trim Data (Disabled)"=w157:u16, "AC Level (1)"=w156:dbl, "Tolerance (10)"=w155:dbl)
            n129 = call "NewtonsPSM_Trim.vi"("AC Level (1)"=w156, "error in"=w154, "Tolerance (10)"=w155, "AC Trim Data (Disabled)"=w157, "VISA.name"=w160) -> ("error out"=w153:errorcluster, "VISA.name out"=w159:refnum<visa-resource-name>)  [unwired: 5 in]
          }
        }
        n130 = call-dynamic "Delacor_lib_QMH_Error Handler - Helper Loop.vi"("Error Debug"=w47, "error in"=w49, "Message Queue in"=w48) -> ()  [unwired: 7 in, 2 out]
      }
      n131 = Unregister For Events(event registration refnum=w30) -> ()  [unwired: 1 in, 1 out]
    }
    frame Error {
      # "Synchronize Caller Events.vi will inform Start Module.vi that the module has launched and will let the code calling Start Module.vi register for broadcasts and would permit the caller receive the broadcast that an error occurred at launch time."
      n132 = call-dynamic "Delacor_lib_QMH_Release Message Queue.vi"("Message Queue"=w374) -> ()  [unwired: 10 in, 1 out]
      n133 = call "Synchronize Caller Events.vi"("Singleton Module Admin in"=w379) -> ("error out"=w376:errorcluster)  [unwired: 9 in, 1 out]
      n134 = call "Module Name--constant.vi"() -> ("Module Name"=w382:string)  [unwired: 11 in]
      n135 = Format Into String(format string="An error occurred during initialization. %s is no longer running.", w382) -> (resulting string=w380:string)  [unwired: 2 in, 1 out]
      n136 = Merge Errors(w378, w376) -> (w377:errorcluster)
      n137 = call "Error Reported.vi"("Additional Information"=w380, "Error"=w377) -> ()  [unwired: 9 in, 1 out]
    }
  }
  n138 = Merge Errors(w18, w25) -> (w17:errorcluster)
  n139 = call "Close Module.vi"("error in (no error)"=w17, "Module Admin in"=w26) -> ("error out"=w20:errorcluster, "External Launch"=w15:bool, "Module Admin out"=w19:refnum<class "Delacor_lib_QMH_Module Admin.lvclass">)  [unwired: 7 in]
  n140 = Unregister For Events(event registration refnum=w24, error in=w20) -> (error out=w16:errorcluster)
  "error out" <- w16
  n141 = case "External Launch?" shown="True" w15 {
    tunnel: w16 -> [_ w388]
    tunnel: w13 -> [_ w387]
    tunnel: w5 -> [_ w385]
    frame False {
    }
    frame True {
      n142 = call-dynamic <vilib>:"Close.vi"("Panel In"=w387) -> ("Error Out"=w386:errorcluster)  [unwired: 10 in]
      n143 = call <vilib>:"Close.vi"("error in (no error)"=w386, "Controller in"=w385) -> ("error out"=w384:errorcluster)  [unwired: 9 in]
      n144 = case shown="Error" w388 {
        tunnel: w384 -> [_ _]
        frame No Error {
        }
        frame Error {
          n145 = disable-structure shown="Default" {
            frame condition #0 (active) {
              n146 = invoke class="VI" method="FP.Open"("Activate"=TRUE ("Activate?")) -> ()  [unwired: 4 in, 5 out]
            }
            frame condition #1 {
              # "Don't show panel on error if running inside a built EXE."
            }
          }
        }
      }
    }
  }
  n147 = local write "Module Admin"(w19) -> ()
